vi "Test IMAQ Image Array to KLB File.vi"() -> ()   [LabVIEW 2012, in "KLB.lvlib"]
doc: "For playing around and testing the Write KLB Stack Function and IMAQ Stack to 1D Array Function\n\nUses a dir full of png files"
uses:
  KLB.lvlib
  VIs/Type Defs/KLB Settings Cluster.ctl
  <vilib>/vision/NI_Vision_Development_Module.lvlib
panel:
  in  "PNG Dir":path=path "C:/Users/FRED/Documents/Projects/KLB/Freds Test Images/Test Images 1"
  out "error out":errorcluster
  out "LineWidth(Pixels)":i32
  out "Y Resolution":i32
  in  "Output Dir":path=path "c:/Test/3.klb"
  in  "KLB Settings":T1={"Logical Cores"=enum."4", "pixelSize"=[1.0, 1.0, 1.0, 1.0, 1.0], "blockSize"=[96, 96, 8, 1, 1], "compressionType"=enum."BZip2", "metadata"=""}
  out "elapsed (ms)":u32
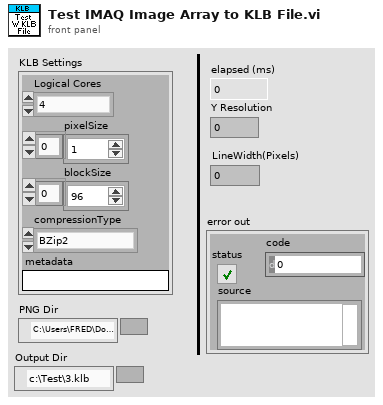
[diagram p1: front panel]
types:
  T1 = typedef "KLB.lvlib/KLB Settings Cluster.ctl" = cluster{"Logical Cores":enum16{"CPU 25%", "CPU 50%", "CPU 75%", "CPU All but 1", "1", "4", "8", "16"}, "pixelSize":sgl[], "blockSize":u32[], "compressionType":enum8{"Uncompressed", "BZip2"}, "metadata":string}
  T2 = enum32{"Map Pixel Pointer", "Unmap Pixel Pointer", "Get Pixels Infos"}
  T3 = typedef "Image Type" = u32
  T4 = typedef "IMAQ Image.ctl" = refnum<image>
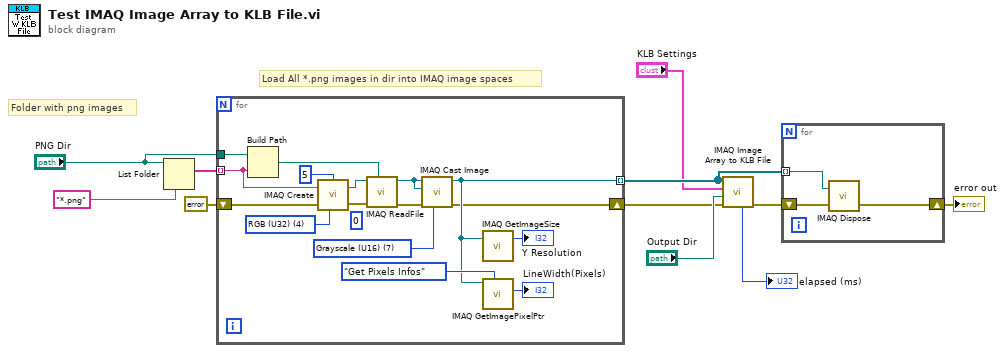
[diagram p0: block diagram]
diagram:
  # "Folder with png images"
  # "Load All *.png images in dir into IMAQ image spaces"
  n1 = List Folder(path="PNG Dir", pattern="*.png") -> (filenames=w10:string[])  [unwired: 2 in, 3 out]
  n2 = for {
    tunnel: w10 -> [w20] mode=indexing
    tunnel: "PNG Dir" -> [w27]
    tunnel: [w13] -> w3 mode=indexing
    shift-right: [w12] -> w5
    shift-left: errorcluster {"status"=FALSE, "code"=0, "source"=""} ("error out") -> [w21]
    (unwired) 0 ("Border Size")
    w19 = T3 7 items=["Grayscale (U8)", "Grayscale (I16)", "Grayscale (SGL)", "Complex (CSG)", "RGB (U32)", "HSL (U32)", "RGB (U64)", "Grayscale (U16)"] ("Image Type")
    w26 = T3 4 items=["Grayscale (U8)", "Grayscale (I16)", "Grayscale (SGL)", "Complex (CSG)", "RGB (U32)", "HSL (U32)", "RGB (U64)", "Grayscale (U16)"] ("Image Type")
    n3 = Build Path(base path=w27, name or relative path=w20) -> (appended path=w23:path)
    n4 = call "IMAQ Create"("Border Size"=5, "Image Name"=w20, "Image Type"=w26, "error in (no error)"=w21) -> ("New Image"=w24:T4, "error out"=w25:errorcluster)  [unwired: 1 in]
    n5 = call "IMAQ ReadFile"("File Path"=w23, "error in (no error)"=w25, "Image"=w24) -> ("error out"=w17:errorcluster, "Image Out"=w18:T4)  [unwired: 4 in, 3 out]
    n6 = call "IMAQ Cast Image"("Image Type"=w19, "error in (no error)"=w17, "Image Dst"=w18, "Image Src"=w18) -> ("error out"=w12:errorcluster, "Image Dst Out"=w13:T4)  [unwired: 6 in]
    n7 = call "IMAQ GetImageSize"("Image"=w13) -> ("Y Resolution"=→"Y Resolution":i32)  [unwired: 3 in, 2 out]
    n8 = call "IMAQ GetImagePixelPtr"("Function"=T2."Get Pixels Infos", "Image"=w13) -> ("LineWidth(Pixels)"=→"LineWidth(Pixels)":i32)  [unwired: 4 in, 5 out]
  }
  n9 = call "IMAQ Image Array to KLB File.vi"("error in (no error)"=w5, "path"="Output Dir", "KLB Settings"="KLB Settings", "Images to Compress"=w3) -> ("error out"=w4:errorcluster, "elapsed (ms)"=→"elapsed (ms)":u32)  [unwired: 6 in]
  n10 = for {
    tunnel: w3 -> [w29] mode=indexing
    shift-right: [w28] -> w1
    shift-left: w4 -> [w30]
    n11 = call "IMAQ Dispose"("Image"=w29, "error in (no error)"=w30) -> ("error out"=w28:errorcluster)  [unwired: 4 in]
  }
  "error out" <- w1
